vi "Initialize.vi"(7 "ChannelName":string="Setpoint.ch%d.SP", 8 "error in":errorcluster, 9 "Number of Channels":u32=1, 10 "Instance Name":string="PluginName", 11 "Setpoint in":refnum<class "Setpoint.lvclass">) -> (0 "error out":errorcluster, 3 "Setpoint out":refnum<class "Setpoint.lvclass">)   [LabVIEW 2023, in "Setpoint.lvclass"]
uses:
  Setpoint.lvclass
  Setpoint.lvclass/Setpoint.ctl
  <vilib>/ADAS Replay HIL/Channels/Tag Wrapper/Polymorphic/Open Consumer Tag (Double).vi
  <vilib>/ADAS Replay HIL/Channels/Tag Wrapper/Polymorphic/Open Consumer Tag (Double).vi/bacb721e-673a-491a-accd-959f2e1f334e.vi
  <vilib>/ADAS Replay HIL/Channels/Tag Wrapper/Polymorphic/Open Consumer Tag (Double).vi/bacb721e-673a-491a-accd-959f2e1f334e.vi/c28b0ead-42ad-4072-80a2-aca7f2bd7ce3.vi
  <vilib>/ADAS Replay HIL/AdasHilServices/AdasHilServices Fill In Error Info Ex.vi
  <vilib>/ADAS Replay HIL/Channels/Tag Wrapper/Tag Wrapper.lvlib
  Utilities/Utilities.lvlib
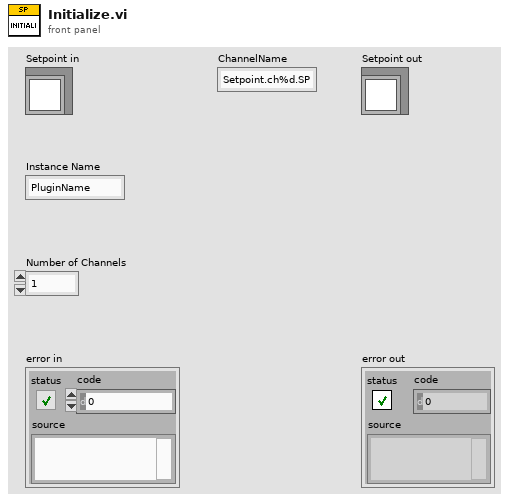
[diagram p1: front panel]
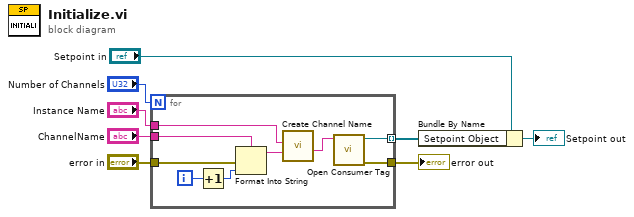
[diagram p0: block diagram]
diagram:
  n1 = for {
    N: "Number of Channels" -> [_]
    tunnel: [w17] -> w8 mode=indexing
    tunnel: [w16] -> w2
    tunnel: "ChannelName" -> [w12]
    tunnel: "Instance Name" -> [w11]
    tunnel: "error in" -> [w13]
    i -> [w15]
    n2 = Increment(x=w15) -> (x+1=w14:i32)
    n3 = Format Into String(format string=w12, error in=w13, w14) -> (resulting string=w10:string)  [unwired: 1 in, 1 out]
    n4 = call "Create Channel Name.vi"("Channel Name"=w10, "Plugin Name"=w11) -> ("Data Channel Name"=w9:string)  [unwired: 8 in, 1 out]
    n5 = call-poly <vilib>:"Open Consumer Tag.vi"("Channel Name"=w9) -> ("error out"=w16:errorcluster, "ADAS HIL Channel"=w17:refnum<k21>)  [unwired: 9 in]
  }
  "error out" <- w2
  n6 = Bundle By Name(cluster="Setpoint in", "Setpoint Object"=w8) -> (→"Setpoint out":refnum<class "Setpoint.lvclass">)
